vi "Speed Indicator.vi"(8 "Reset Encoder 0":bool, 9 "Speed M2":dbl(slide) scale=-1.0..1.0, 10 "Speed M1 2":dbl(slide) scale=-1.0..1.0, 11 "Speed M0":dbl(slide) scale=-1.0..1.0) -> (0 "Speed M2":dbl, 1 "Speed M1":dbl, 2 "Speed M0":dbl, 3 "Distance M2":dbl, 4 "Distance M1":dbl, 5 "Distance M0":dbl)   [LabVIEW 2018]
panel:
  in  "Boolean":bool
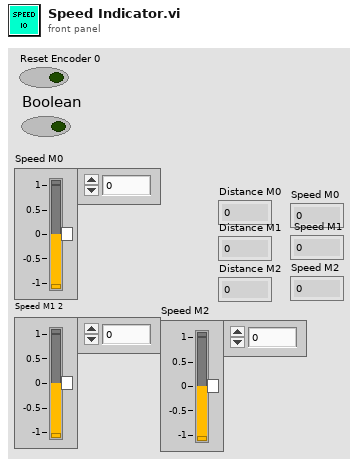
[diagram p1: front panel]
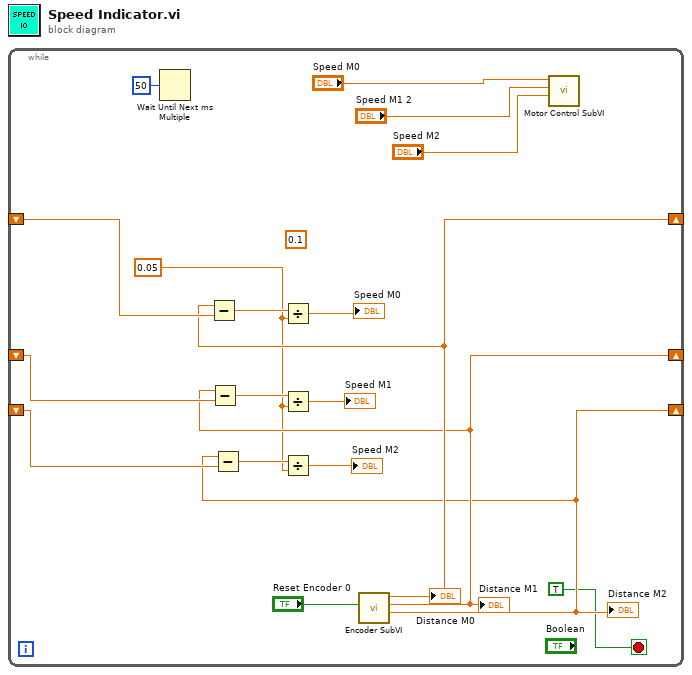
[diagram p0: block diagram]
diagram:
  n1 = while {
    shift-right: [w12] -> _
    shift-left: _ -> [w19]
    shift-right: [w9] -> _
    shift-left: _ -> [w11]
    shift-right: [w8] -> _
    shift-left: _ -> [w10]
    stop <- TRUE stop-if-true
    (unwired) 0.1 ("y")
    w5 = 0.05 ("Delay Time (s)")
    n2 = Wait Until Next ms Multiple(millisecond multiple=u32 50) -> ()  [unwired: 1 out]
    n3 = call "Encoder SubVI.vi"("Reset Encoders"="Reset Encoder 0") -> ("Distance M2"=w8:dbl, "Distance M1"=w9:dbl, "Distance M0"=w12:dbl)  [unwired: 7 in, 1 out]
    "Distance M0" <- w12
    "Distance M1" <- w9
    "Distance M2" <- w8
    n4 = Subtract(x=w12, y=w19) -> (x-y=w18:dbl)
    n5 = Subtract(x=w9, y=w11) -> (x-y=w16:dbl)
    n6 = Subtract(x=w8, y=w10) -> (x-y=w15:dbl)
    n7 = Divide(x=w18, y=w5) -> (x/y=→"Speed M0":dbl)
    n8 = Divide(x=w16, y=w5) -> (x/y=→"Speed M1":dbl)
    n9 = Divide(x=w15, y=w5) -> (x/y=→"Speed M2":dbl)
    n10 = call "Motor Control SubVI.vi"("Speed M2"="Speed M2", "Speed M1"="Speed M1 2", "Speed M0"="Speed M0") -> ()  [unwired: 8 in, 1 out]
  }
